vi "ZIDevice_SetParameters(Values).vi"(8 "error in (no error)":errorcluster, 10 "Parameters":T1[](array[typedef]) {"Value" format="%#_6p"}, 11 "Handle In":T2 {"Handle" format="0x%08x"; "Conn" format="0x%08x"}) -> (0 "error out":errorcluster, 3 "Handle Out":T2 {"Handle" format="0x%08x"; "Conn" format="0x%08x"})   [LabVIEW 2016, in "General.lvlib"]
uses:
  General.lvlib
  <instrlib>/Zurich Instruments LabOne/Public/ziTypeHandle.ctl
  Ctl_SetParameter(Value).ctl
  <instrlib>/Zurich Instruments LabOne/Public/Configure/ziSetValueDoubleArray.vi
  <instrlib>/Zurich Instruments LabOne/Zurich Instruments LabOne.lvlib
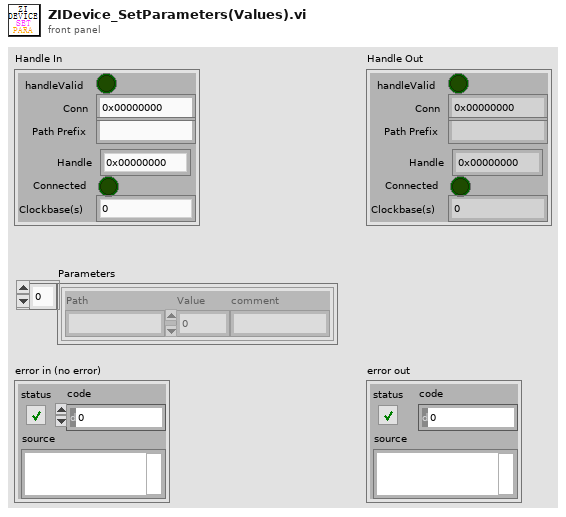
[diagram p1: front panel]
types:
  T1 = typedef "General.lvlib/Ctl_SetParameter(Value).ctl" = cluster{"Path":string, "Value":dbl, "comment":string}
  T2 = typedef "Zurich Instruments LabOne.lvlib/ziTypeHandle.ctl" = cluster{"handleValid":bool, "Conn":u64, "Path Prefix":string, "Handle":u64, "Connected":bool, "Clockbase(s)":dbl}
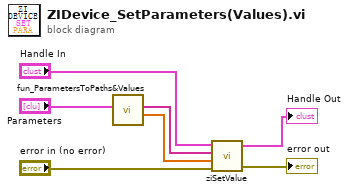
[diagram p0: block diagram]
diagram:
  n1 = call "fun_ParametersToPaths&Values.vi"("Parameters"="Parameters") -> ("Values"=w1:dbl[], "Paths"=w2:string[])  [unwired: 9 in]
  n2 = call-poly <instrlib>:"ziSetValue.vi"("Error In"="error in (no error)", "Values"=w1, "Paths"=w2, "Handle In"="Handle In") -> ("Error Out"=→"error out":errorcluster, "Handle Out"=→"Handle Out":T2)  [unwired: 1 in]
